vi "Konstant 0-100 hinzufuegen.vi"(10 "Signalverläufe":T1) -> (2 "Signalverläufe":T1)   [LabVIEW 2020, in "Gaszuordnung AO.lvlib"]
uses:
  Gaszuordnung AO.lvlib
  FT-IR/TOOLweb Interface Library/TOOLweb Signalverlaeufe.ctl
  FT-IR/TOOLweb Interface Library/TOOLweb Interface Hilfs-VIs.lvlib
  FT-IR/TOOLweb Interface Library/Typdefinitionen.lvlib
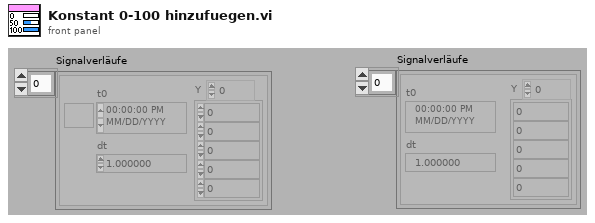
[diagram p1: front panel]
types:
  T1 = typedef "FT-IR.lvlib/TOOLweb Interface.lvlib/Typdefinitionen.lvlib/TOOLweb Signalverlaeufe.ctl" = waveform(dbl)[]
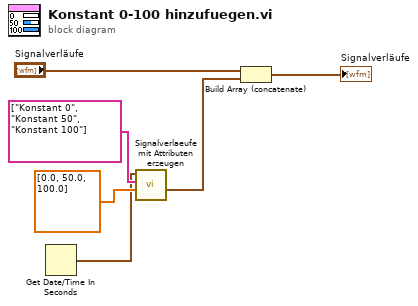
[diagram p0: block diagram]
diagram:
  n1 = Get Date/Time In Seconds() -> (seconds since 1Jan1904=w1:timestamp)
  n2 = call "Signalverlaeufe mit Attributen erzeugen.vi"("Messwerte"=dbl[] [0.0, 50.0, 100.0], "Namen"=string[] ["Konstant 0", "Konstant 50", "Konstant 100"], "Zeitstempel"=w1) -> ("Signalverläufe"=w6:waveform(dbl)[])  [unwired: 8 in]
  n3 = Build Array (concatenate)("Signalverläufe", w6) -> (→"Signalverläufe":T1)
